vi "Write t.vi"(8 "error in (no error)":errorcluster, 10 "t":dbl, 11 "Sync Time MSG in":refnum<class "Sync Time MSG.lvclass">) -> (0 "error out":errorcluster, 3 "Sync Time MSG out":refnum<class "Sync Time MSG.lvclass">)   [LabVIEW 2017, in "Controller.lvlib" / "Sync Time MSG.lvclass"]
uses:
  Sync Time MSG.lvclass
  Sync Time MSG.lvclass/Sync Time MSG.ctl
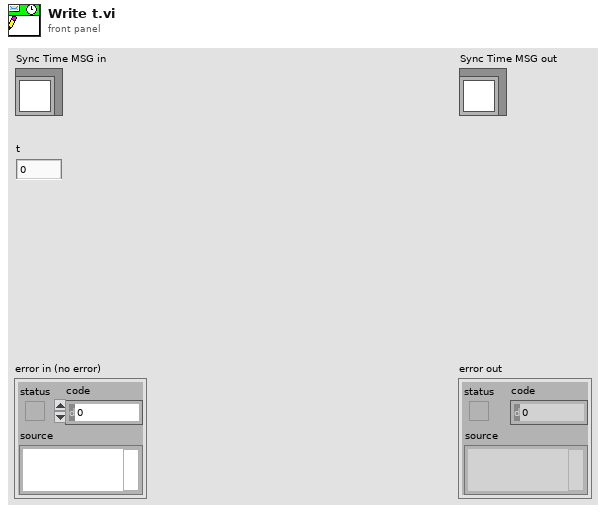
[diagram p1: front panel]
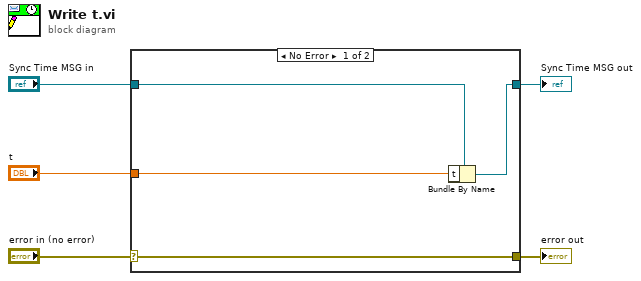
[diagram p0: block diagram]
diagram:
  n1 = case shown="No Error" "error in (no error)" {
    selector: "error in (no error)" -> [w9 w10]
    tunnel: [w9 w10] -> w4
    tunnel: [w7 w11] -> w2
    tunnel: "Sync Time MSG in" -> [w8 w11]
    tunnel: "t" -> [w6 _]
    frame No Error {
      n2 = Bundle By Name(cluster=w8, "t"=w6) -> (w7:refnum<class "Sync Time MSG.lvclass">)
    }
    frame Error {
    }
  }
  "error out" <- w4
  "Sync Time MSG out" <- w2
